vi "Crop (Rectangle Points Greyscale).vi"(6 "Point B":T1, 8 "error in (no error)":errorcluster, 9 "Point A":T2, 10 "Greyscale Image Destination in":T3, 11 "Greyscale Image Source in":T3) -> (0 "error out":errorcluster, 1 "Computed Size":T1, 3 "Greyscale Image Destination":T3)   [LabVIEW 2020, in "image.lvlib"]
doc: "Crop the Source Image region specified by two corner points into the Destination Image."
uses:
  image.lvlib
  Greyscale Image.ctl
  common/Image Point (Float).ctl
  common/Image Point (Integer).ctl
  2dc01dea-48f6-4df4-8727-934e95e7e307.vi
  <vilib>/Utility/error.llb/Error Cluster From Error Code.vi
  common/common.lvlib
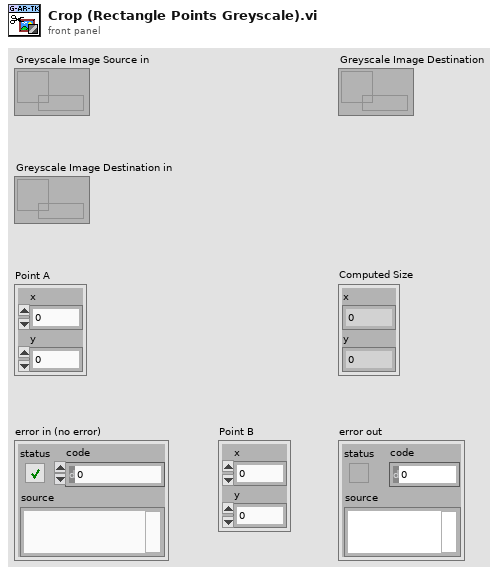
[diagram p1: front panel]
types:
  T1 = typedef "common.lvlib/Image Point (Float).ctl" = cluster{"x":dbl, "y":dbl}
  T2 = typedef "common.lvlib/Image Point (Integer).ctl" = cluster{"x":i32, "y":i32}
  T3 = typedef "image.lvlib/Greyscale Image.ctl" = refnum<data-value>
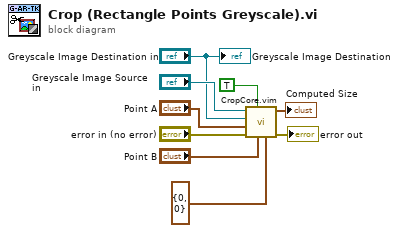
[diagram p0: block diagram]
diagram:
  n1 = call "CropCore.vim"("Other Point"=T2 {"x"=0, "y"=0}, "Size"="Point B", "Use Size"=TRUE, "error in (no error)"="error in (no error)", "Origin"="Point A", "Dst"="Greyscale Image Destination in", "Src"="Greyscale Image Source in") -> ("error out"=→"error out":errorcluster, "Computed Size"=→"Computed Size":T1)  [unwired: 3 in]
  "Greyscale Image Destination" <- "Greyscale Image Destination in"
